vi "TCP-error-definitions.vi"() -> (4 "Descriptions":string[](array[string])=["AccessDenied: TCP/IP networking access was denied.", "Communications: TCP/IP network communications error occured.", "NotConnected: Client is not connected to the server.", "IllegalClientId: Internal error.", "InvalidPersistState: Internal error.", "ServerNameNotFound: Requested server name is not valid.", "InvalidParameter: Bad parameter to a method call.", "Network: TCP/IP networking error.", "DataNotFound: Requested data file not found.", "PathNotFound: Specified path does not exist.", "Access: Access to server file system was denied.", "LocalAccess: Access to the client file system was denied or Server is under control of a local pendant.", "DataUnknown: XML data type is unknown.", "EventHandling: Internal event processing error.", "NotAvailable: Server is not currently available.", "Aborting: Server is currently aborting.", "Aborted: Server action was aborted.", "Exception: Internal error.", "Timeout: Requested action timed out.", "NoData: Thre requested fixed data was empty.", "DataExists: Destination file already exists and over-write not specified.", "RemoteAccess: Server is already connected to a client.", "StateError: Server is in error state and unavailable.", "BufferFull: Streaming data transmit buffer is full."], 6 "Error codes":i32[](array[numeric]))   [LabVIEW 2013, in "EC1000-control.lvlib" / "SM1000-control.lvclass"]
uses:
  SM1000-control.lvclass
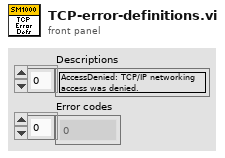
[diagram p1: front panel]
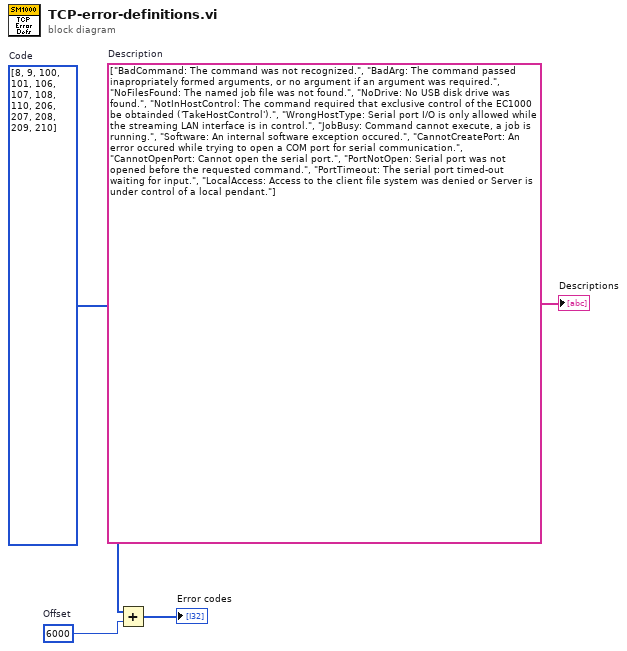
[diagram p0: block diagram]
diagram:
  w4 = 6000  # Offset
  w3 = i32[] [8, 9, 100, 101, 106, 107, 108, 110, 206, 207, 208, 209, 210]  # Code
  w2 = string[] ["BadCommand: The command was not recognized.", "BadArg: The command passed inapropriately formed arguments, or no argument if an argument was required.", "NoFilesFound: The named job file was not found.", "NoDrive: No USB disk drive was found.", "NotInHostControl: The command required that exclusive control of the EC1000 be obtainded ('TakeHostControl').", "WrongHostType: Serial port I/O is only allowed while the streaming LAN interface is in control.", "JobBusy: Command cannot execute, a job is running.", "Software: An internal software exception occured.", "CannotCreatePort: An error occured while trying to open a COM port for serial communication.", "CannotOpenPort: Cannot open the serial port.", "PortNotOpen: Serial port was not opened before the requested command.", "PortTimeout: The serial port timed-out waiting for input.", "LocalAccess: Access to the client file system was denied or Server is under control of a local pendant."]  # Description
  n1 = Add(x=w3, y=w4) -> (x+y=→"Error codes":i32[])
  "Descriptions" <- w2
